vi "sensor_Module.vi"(8 "error in (no error)":errorcluster) -> (0 "error out":errorcluster)   [LabVIEW 2013]
doc: "This is the sensor module, it sends the location of the elevator to the controller. It initilizes and shuts down. \n [Covers: UI4]"
uses:
  Messaging/Msg_Control.ctl
  Sensor_Enum.ctl
  Sensor_Station.ctl
panel:
  in  "Elevator Position":T1 scale=0.0..3.0
  # "[Covers: UI4]"
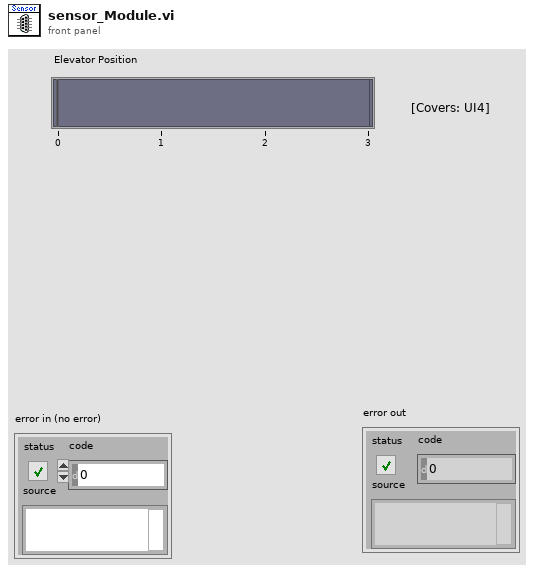
[diagram p1: front panel]
types:
  T1 = typedef "Sensor_Station.ctl" = u8
  T2 = typedef "Sensor_Enum.ctl" = enum16{"Init", "Idle", "Send_Position", "Terminate"}
  T3 = typedef "Msg_Control.ctl" = enum16{"Init_Msg", "Sent_Inits", "Get_Ref", "Close_Ref"}
  T4 = cluster{"queue out":refnum<queue>, "queue out":refnum<queue>, "queue out":refnum<queue>}
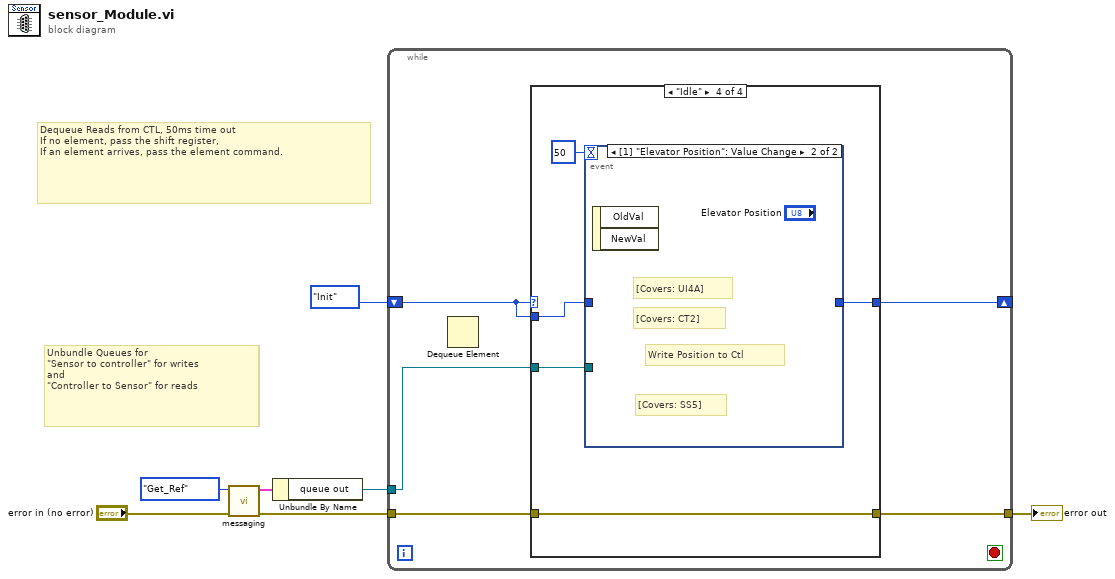
[diagram p0: block diagram]
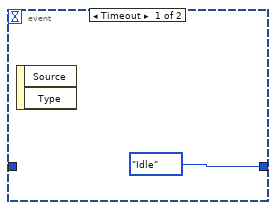
[diagram p5: hidden frame]
diagram:
  # "Unbundle Queues for\n\"Sensor to controller\" for writes\nand\n\"Controller to Sensor\" for reads"
  # "Dequeue Reads from CTL, 50ms time out\nIf no element, pass the shift register,\nIf an element arrives, pass the element command."
  # "Unbundle Queues for\n\"Sensor to controller\" for writes\nand\n\"Controller to Sensor\" for reads"
  n1 = call "messaging.vi"("error in (no error)"="error in (no error)", "Message_Control"=Msg_Control."Get_Ref") -> ("error out"=w3:errorcluster, "REfs Out"=w2:T4)  [unwired: 8 in]
  n2 = Unbundle By Name(w2) -> ("queue out"=w1:refnum<queue>)
  n3 = while {
    tunnel: [w12] -> w7
    tunnel: w3 -> [w11]
    shift-right: [w10] -> _
    shift-left: Sensor_Enum."Init" ("Sensor_Enum") -> [w9]
    tunnel: w1 -> [w8]
    stop <- _ stop-if-true
    n4 = Dequeue Element() -> ()  [unwired: 3 in, 4 out]
    n5 = case shown="\"Idle\"" w9 {
      tunnel: [w14 w16 w18 w23] -> w12
      tunnel: w11 -> [w14 w16 w18 w23]
      tunnel: [w13 w15 w17 w21] -> w10
      tunnel: w9 -> [w13 w15 w17 w22]
      tunnel: w8 -> [_ _ _ w19]
      frame "Init", Default {
        # "[Covers: IS3]"
        # "Set Sensor to zero position"
        # "1st queu element is Init, from msg handler"
      }
      frame "Terminate" {
        # "[Covers: TS1]\n[Covers: TS2]"
        # "Disable Sensor\nEnd the loop"
        # "End loop, implement terminate requirements"
      }
      frame "Send_Position" {
        # "Not Used"
      }
      frame "Idle" {
        n6 = event shown="[1] \"Elevator Position\": Value Change" {
          selector: _ -> [_ _]
          dyn-events: _ -> [_ _]
          timeout: 50 -> [_ _]
          tunnel: w22 -> [_ _]
          tunnel: [Sensor_Enum."Idle" ("Sensor_Enum 2") _] -> w21
          tunnel: w19 -> [_ _]
          event Timeout {
            n7 = event-data() -> ()  [unwired: 1 in, 2 out]
          }
          event Value Change {
            # "[Covers: SS5]"
            # "[Covers: UI4A]"
            # "[Covers: CT2]"
            # "Write Position to Ctl"
            n8 = event-data() -> ()  [unwired: 1 in, 2 out]
          }
        }
      }
    }
  }
  "error out" <- w7
